vi "5492_WPI_RobotDriveOpen4MotorWithTalonSRX_Position.vi"(0 "Front Left Motor":T1=enum."Invalid", 1 "Front Left Motor Inverted":bool, 2 "Current Limit (Amps)":dbl=100.0 format="%#_13g", 3 "Front Right Motor Inverted":bool, 5 "Front Right Motor":T1=enum."Invalid", 7 "Back Left Motor":T1=enum."Invalid", 9 "Back Right Motor":T1=enum."Invalid", 11 "error in (no error)":errorcluster, 12 "Back Left Motor Inverted":bool, 13 "Ramp Time (s)":dbl=0.5 format="%#_13g", 14 "Back Right Motor Inverted":bool) -> (4 "RobotDriveDevRef":T2={"DevStatus"={"status"=FALSE, "code"=0, "source"=""}, "Motors[]"=[], "Square Inputs"=FALSE, "Max Output"=1.0}, 15 "error out":errorcluster)   [LabVIEW 2017]
doc: "Opens a reference to the robot drive for a two-motor robot using TalonSRX motor controllers.\n\nThis software is licensed. Open the labview\\readme\\WPI Robotics Library Open Source License.txt file for more information."
uses:
  <vilib>/Rock Robotics/SystemInterfaces/DIO/FPGA_DIOPWMChannel.ctl
  <vilib>/Rock Robotics/WPI/RobotDrive/WPI_RobotDriveDevRef.ctl
  <vilib>/Rock Robotics/WPI/MotorControl/WPI_MotorControlDeviceRef.ctl
  <vilib>/Rock Robotics/WPI/MotorControl/WPI_MotorControlType.ctl
  <vilib>/Rock Robotics/WPI/PWM/WPI_PWMDeadband.ctl
  <vilib>/Rock Robotics/SystemInterfaces/DIO/FPGA_DIOChannel.ctl
  <vilib>/Rock Robotics/WPI/SafetyOutput/WPI_SafetyOutputConfigMenu.ctl
  Public/Documents/Cross The Road Electronics/Phoenix-LabVIEW/Motor Controller/Controls/CTRE_Phoenix_MotorControl_ControlMode.ctl
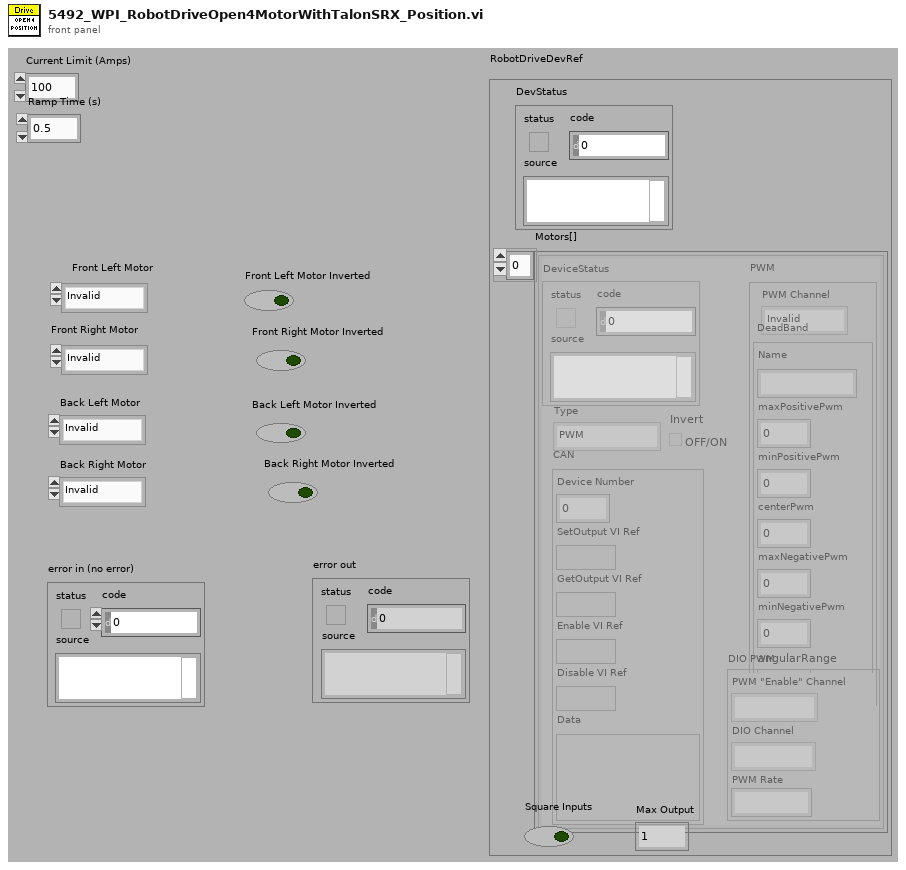
[diagram p1: front panel]
types:
  T1 = typedef "FPGA_DIOPWMChannel.ctl" = enum8{"PWM 0", "PWM 1", "PWM 2", "PWM 3", "PWM 4", "PWM 5", "PWM 6", "PWM 7", "PWM 8", "PWM 9", "PWM MXP 0", "PWM MXP 1", "PWM MXP 2", "PWM MXP 3", "PWM MXP 4", "PWM MXP 5", "PWM MXP 6", "PWM MXP 7", "PWM MXP 8", "PWM MXP 9", "Invalid"}
  T2 = typedef "WPI_RobotDriveDevRef.ctl" = cluster{"DevStatus":errorcluster, "Motors[]":T3[], "Square Inputs":bool, "Max Output":dbl}
  T3 = typedef "WPI_MotorControlDeviceRef.ctl" = cluster{"DeviceStatus":errorcluster, "Type":T4, "PWM":cluster{"PWM Channel":T1, "DeadBand":T5}, "CAN":cluster{"Device Number":u8, "SetOutput VI Ref":variant, "GetOutput VI Ref":variant, "Enable VI Ref":variant, "Disable VI Ref":variant, "Data":variant}, "Invert":bool, "DIO PWM":cluster{"PWM \"Enable\" Channel":T1, "DIOChannel":T6, "PWM Rate":dbl}}
  T4 = typedef "WPI_MotorControlType.ctl" = enum16{"PWM", "CAN", "DIO PWM"}
  T5 = typedef "WPI_PWMDeadband.ctl" = cluster{"Name":string, "maxPositivePwm":i32, "minPositivePwm":i32, "centerPwm":i32, "maxNegativePwm":i32, "minNegativePwm":i32, "angularRange":u16}
  T6 = typedef "FPGA_DIOChannel.ctl" = enum8{"DIO 0", "DIO 1", "DIO 2", "DIO 3", "DIO 4", "DIO 5", "DIO 6", "DIO 7", "DIO 8", "DIO 9", "DIO MXP 0", "DIO MXP 1", "DIO MXP 2", "DIO MXP 3", "DIO MXP 4", "DIO MXP 5", "DIO MXP 6", "DIO MXP 7", "DIO MXP 8", "DIO MXP 9", "DIO MXP 10", "DIO MXP 11", "DIO MXP 12", "DIO MXP 13", "DIO MXP 14", "DIO MXP 15", "SPI Port CS1", "SPI Port CS2", "SPI Port CS3", "SPI Port MISO", "SPI Port MOSI", "Invalid"}
  T7 = typedef "WPI_SafetyOutputConfigMenu.ctl" = enum16{"Enable", "Disable"}
  T8 = typedef "CTRE_Phoenix_MotorControl_ControlMode.ctl" = u16
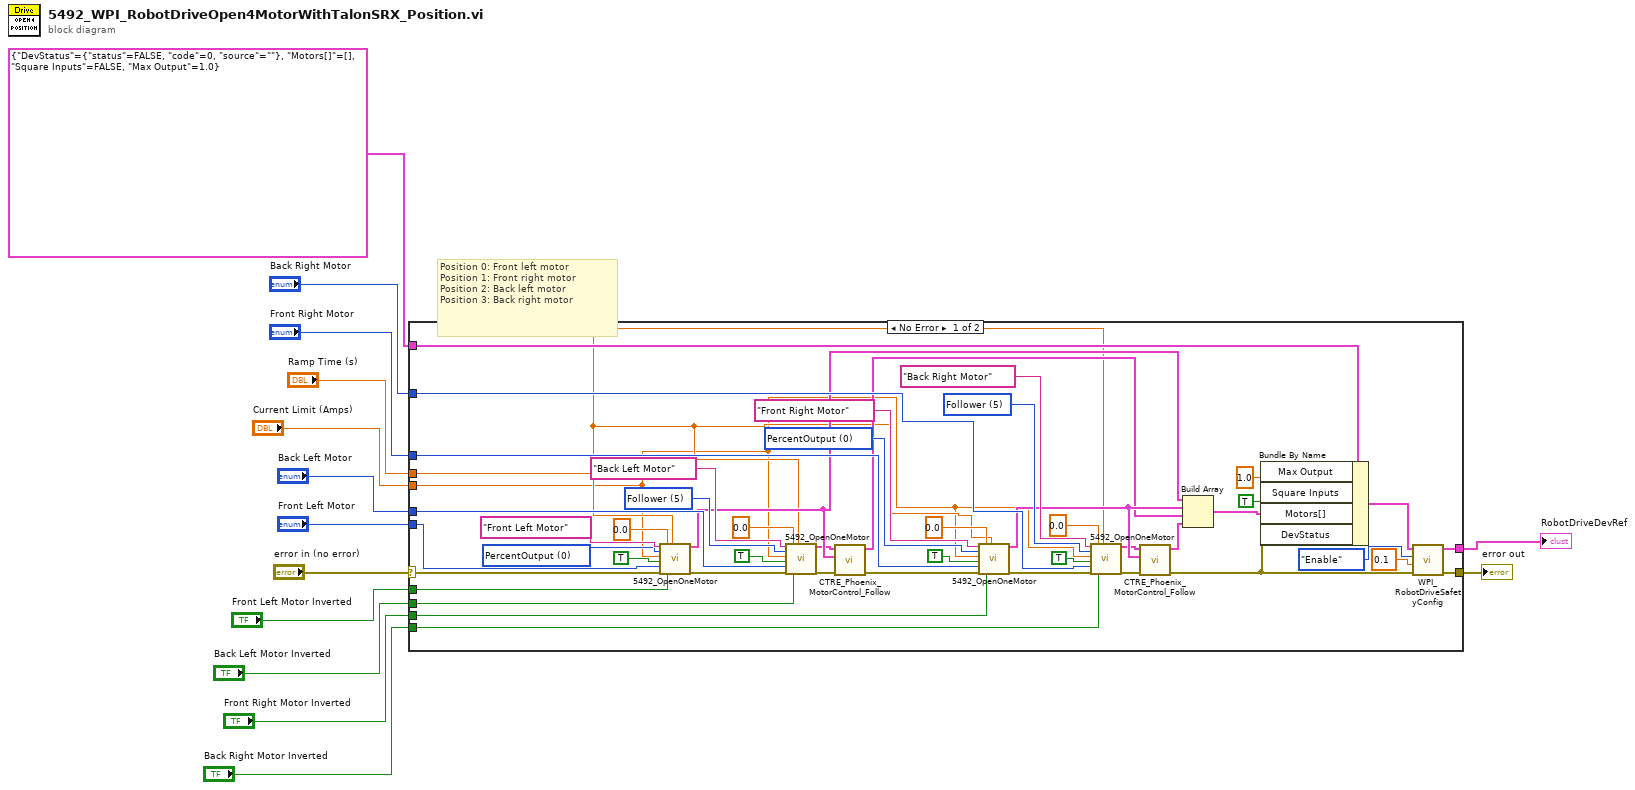
[diagram p0: block diagram]
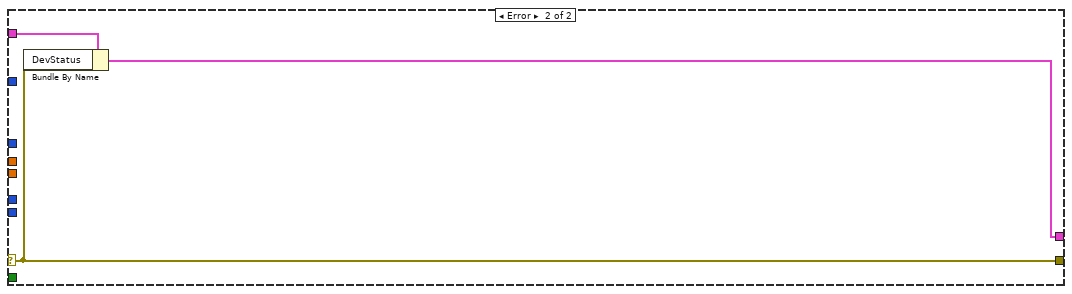
[diagram p2: hidden frame]
diagram:
  # "Position 0: Front left motor\nPosition 1: Front right motor\nPosition 2: Back left motor\nPosition 3: Back right motor"
  n1 = case shown="No Error" "error in (no error)" {
    selector: "error in (no error)" -> [w23 w63]
    tunnel: "Front Left Motor" -> [w52 _]
    tunnel: "Front Right Motor" -> [w53 _]
    tunnel: [w56 w65] -> w7
    tunnel: "Front Left Motor Inverted" -> [w47 _]
    tunnel: "Front Right Motor Inverted" -> [w46 _]
    tunnel: T2 {"DevStatus"={"status"=FALSE, "code"=0, "source"=""}, "Motors[]"=[], "Square Inputs"=FALSE, "Max Output"=1.0} ("RobotDriveDevRef") -> [w61 w64]
    tunnel: [w57 w63] -> w9
    tunnel: "Back Left Motor" -> [w51 _]
    tunnel: "Back Right Motor" -> [w50 _]
    tunnel: "Back Left Motor Inverted" -> [w48 _]
    tunnel: "Back Right Motor Inverted" -> [w49 _]
    tunnel: "Ramp Time (s)" -> [w16 _]
    tunnel: "Current Limit (Amps)" -> [w15 _]
    frame No Error {
      w38 = T8 0 items=["PercentOutput"=0, "Position"=1, "Velocity"=2, "Current"=3, "Follower"=5, "MotionProfile"=6, "MotionMagic"=7, "MotionMagicArc"=8, "MotionProfileArc"=10, "Disabled"=15] ("Control Mode")
      w39 = T8 0 items=["PercentOutput"=0, "Position"=1, "Velocity"=2, "Current"=3, "Follower"=5, "MotionProfile"=6, "MotionMagic"=7, "MotionMagicArc"=8, "MotionProfileArc"=10, "Disabled"=15] ("Control Mode")
      w40 = T8 5 items=["PercentOutput"=0, "Position"=1, "Velocity"=2, "Current"=3, "Follower"=5, "MotionProfile"=6, "MotionMagic"=7, "MotionMagicArc"=8, "MotionProfileArc"=10, "Disabled"=15] ("Control Mode")
      w41 = T8 5 items=["PercentOutput"=0, "Position"=1, "Velocity"=2, "Current"=3, "Follower"=5, "MotionProfile"=6, "MotionMagic"=7, "MotionMagicArc"=8, "MotionProfileArc"=10, "Disabled"=15] ("Control Mode")
      n2 = call "5492_OpenOneMotor.vi"("refnum name"="Front Left Motor", "Control Mode"=w38, "Current Limit (Amps)"=w15, "Current Limit?"=TRUE, "Device Number"=w52, "error in"=w23, "Output"=0.0, "Invert"=w47, "Ramp Time (s)"=w16) -> ("MotorControlDevRef"=w37:T3, "error out"=w22:errorcluster)  [unwired: 9 in]
      n3 = call "5492_OpenOneMotor.vi"("refnum name"="Back Left Motor", "Control Mode"=w41, "Current Limit (Amps)"=w15, "Current Limit?"=TRUE, "Device Number"=w51, "error in"=w22, "Output"=0.0, "Invert"=w48, "Ramp Time (s)"=w16) -> ("MotorControlDevRef"=w33:T3, "error out"=w19:errorcluster)  [unwired: 9 in]
      n4 = call "CTRE_Phoenix_MotorControl_Follow.vi"("error in (no error)"=w19, "Master Controller to Follow"=w37, "PhoenixMotorControlDevRef"=w33) -> ("error out"=w18:errorcluster, "PhoenixMotorControlDevRef"=w35:T3)  [unwired: 7 in]
      n5 = call "5492_OpenOneMotor.vi"("refnum name"="Front Right Motor", "Control Mode"=w39, "Current Limit (Amps)"=w15, "Current Limit?"=TRUE, "Device Number"=w53, "error in"=w18, "Output"=0.0, "Invert"=w46, "Ramp Time (s)"=w16) -> ("MotorControlDevRef"=w36:T3, "error out"=w21:errorcluster)  [unwired: 9 in]
      n6 = call "5492_OpenOneMotor.vi"("refnum name"="Back Right Motor", "Control Mode"=w40, "Current Limit (Amps)"=w15, "Current Limit?"=TRUE, "Device Number"=w50, "error in"=w21, "Output"=0.0, "Invert"=w49, "Ramp Time (s)"=w16) -> ("MotorControlDevRef"=w32:T3, "error out"=w17:errorcluster)  [unwired: 9 in]
      n7 = call "CTRE_Phoenix_MotorControl_Follow.vi"("error in (no error)"=w17, "Master Controller to Follow"=w36, "PhoenixMotorControlDevRef"=w32) -> ("error out"=w20:errorcluster, "PhoenixMotorControlDevRef"=w34:T3)  [unwired: 7 in]
      n8 = Build Array(w37, w36, w35, w34) -> (w62:T3[])
      n9 = Bundle By Name(cluster=w61, "Max Output"=1.0, "Square Inputs"=TRUE, "Motors[]"=w62, "DevStatus"=w20) -> (w59:T2)
      n10 = call <vilib>:"WPI_RobotDriveSafetyConfig.vi"("error in (no error)"=w20, "timeout (s)"=0.1, "mode"=WPI_SafetyOutputConfigMenu."Enable", "RobotDriveDevRef"=w59) -> ("error out"=w57:errorcluster, "RobotDriveDevRef"=w56:T2)  [unwired: 6 out]
    }
    frame Error {
      n11 = Bundle By Name(cluster=w64, "DevStatus"=w63) -> (w65:T2)
    }
  }
  "RobotDriveDevRef" <- w7
  "error out" <- w9
